vi "munmap.vi"(8 "error in (no error)":errorcluster, 10 "size (bytes)":u64, 11 "pointer":u64) -> (0 "error out":errorcluster)   [LabVIEW 2013, in "Shared Memory.lvlib" / "Shared Memory.lvclass"]
doc: "Wrapper VI for Linux function munmap()."
uses:
  Shared Memory.lvclass
  Controls/functions.ctl
  <vilib>/NI/NI Linux RT Errno/Linux Errno.lvlib
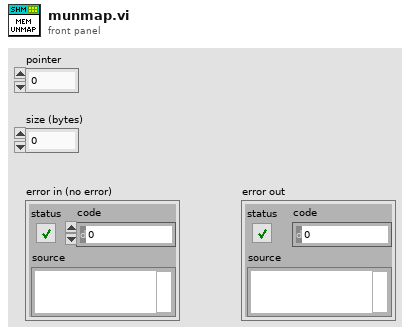
[diagram p1: front panel]
types:
  T1 = typedef "Shared Memory.lvlib/Shared Memory.lvclass/functions.ctl" = enum16{"unspecified", "shm_open", "ftruncate", "mmap", "munmap", "close", "shm_unlink", "fstat"}
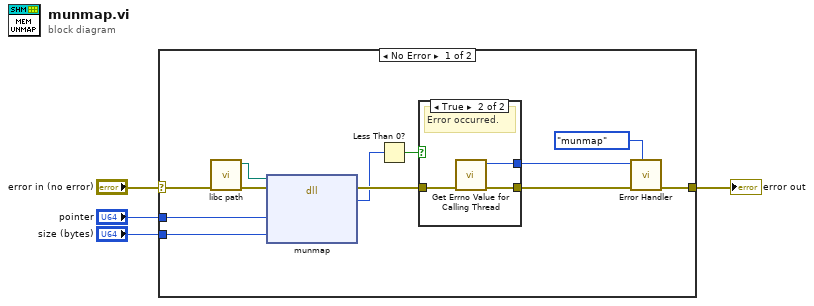
[diagram p0: block diagram]
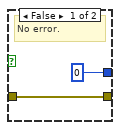
[diagram p2: hidden frame]
diagram:
  n1 = case shown="No Error" "error in (no error)" {
    selector: "error in (no error)" -> [w13 w22]
    tunnel: [w14 w22] -> w4
    tunnel: "pointer" -> [w12 _]
    tunnel: "size (bytes)" -> [w11 _]
    frame No Error {
      n2 = call "libc path.vi"("error in (no error)"=w13) -> ("error out"=w9:errorcluster, "path to libc"=w8:path)  [unwired: 9 in]
      n3 = dll-call lib="?" fn="munmap"(path in=w8, error in=w9, "addr"=w12, "size"=w11) -> (error out=w7:errorcluster, "status"=w5:i32)  [unwired: 3 in, 1 out]
      n4 = Less Than 0?(x=w5) -> (x < 0?=w6:bool)
      n5 = case shown="True" w6 {
        tunnel: w7 -> [w18 w21]
        tunnel: [w18 w20] -> w15
        tunnel: [0 ("errno") w19] -> w10
        frame False {
          # "No error."
        }
        frame True {
          # "Error occurred."
          n6 = call <vilib>:"Get Errno Value for Calling Thread.vi"("error in (no error)"=w21) -> ("error out"=w20:errorcluster, "errno"=w19:i32)  [unwired: 9 in]
        }
      }
      n7 = call "Error Handler.vi"("function"=functions."munmap", "error in (no error)"=w15, "errno"=w10) -> ("error out"=w14:errorcluster)  [unwired: 8 in]
    }
    frame Error {
    }
  }
  "error out" <- w4
